vi "Init Sync Stuff.vi"(8 "error in (no error)":errorcluster, 10 "Barometer Bricklet in":refnum<class "Barometer Bricklet.lvclass">) -> (0 "error out":errorcluster, 2 "Barometer Bricklet out":refnum<class "Barometer Bricklet.lvclass">)   [LabVIEW 2011, in "Tinkerforge.lvlib" / "Barometer Bricklet.lvclass"]
doc: "This VI is the child implementation of \"Init Sync Stuff.vi\" and initializes all synchronization objects of this child object."
uses:
  Barometer Bricklet.lvclass
  Barometer Bricklet.lvclass/Barometer Bricklet.ctl
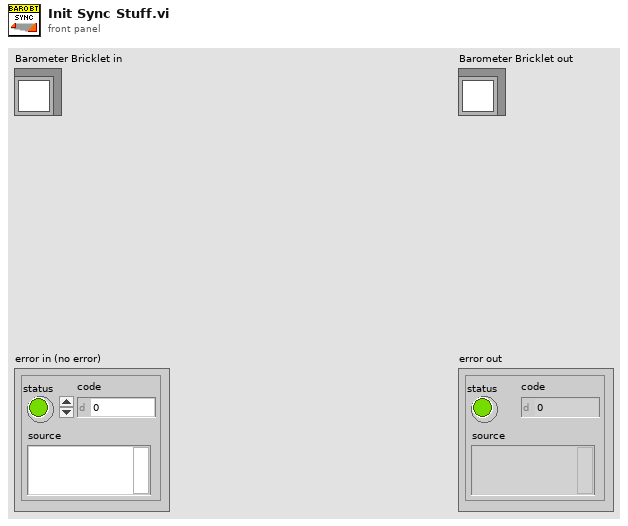
[diagram p1: front panel]
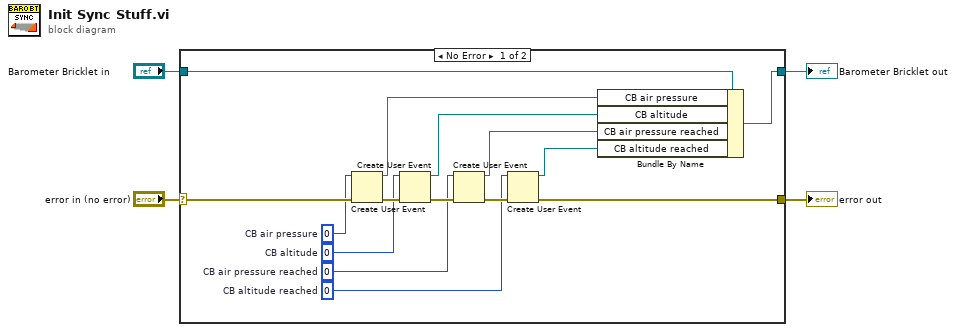
[diagram p0: block diagram]
diagram:
  n1 = case shown="No Error" "error in (no error)" {
    selector: "error in (no error)" -> [w17 w20]
    tunnel: "Barometer Bricklet in" -> [w19 w21]
    tunnel: [w9 w20] -> w2
    tunnel: [w18 w21] -> w1
    frame No Error {
      w10 = 0  # CB altitude reached
      w11 = 0  # CB air pressure reached
      w12 = 0  # CB altitude
      w16 = 0  # CB air pressure
      n2 = Create User Event(user event datatype=w16, error in=w17) -> (user event=w8:refnum<user-event>, error out=w15:errorcluster)
      n3 = Create User Event(user event datatype=w12, error in=w15) -> (user event=w7:refnum<user-event>, error out=w14:errorcluster)
      n4 = Create User Event(user event datatype=w11, error in=w14) -> (user event=w6:refnum<user-event>, error out=w13:errorcluster)
      n5 = Create User Event(user event datatype=w10, error in=w13) -> (user event=w5:refnum<user-event>, error out=w9:errorcluster)
      n6 = Bundle By Name(cluster=w19, "CB air pressure"=w8, "CB altitude"=w7, "CB air pressure reached"=w6, "CB altitude reached"=w5) -> (w18:refnum<class "Barometer Bricklet.lvclass">)
    }
    frame Error {
    }
  }
  "error out" <- w2
  "Barometer Bricklet out" <- w1
